vi "DHE_DRV_stop_sequence.vi"(11 "error in (no error)":errorcluster) -> (15 "error out":errorcluster)   [LabVIEW 2016]
doc: "This VI closes the I/O interface with the instrument."
uses:
  c/lib/libarcDHE.so
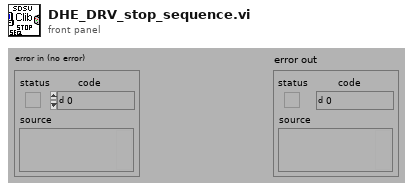
[diagram p1: front panel]
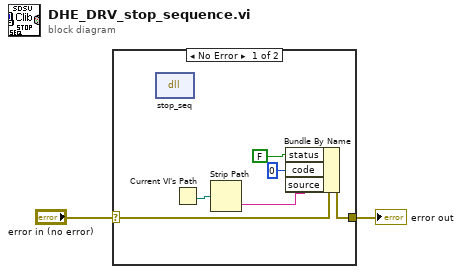
[diagram p0: block diagram]
diagram:
  n1 = case shown="No Error" "error in (no error)" {
    selector: "error in (no error)" -> [w5 w9]
    tunnel: [w6 w9] -> w2
    frame No Error {
      n2 = dll-call lib="home/simager/panview/PAN/Modules/SDSU/private/c/lib/libarcDHE.so" fn="stop_seq"() -> ()  [unwired: 3 in, 3 out]
      n3 = Current VI's Path() -> (path=w8:path)
      n4 = Strip Path(path=w8) -> (name=w7:string)  [unwired: 1 out]
      n5 = Bundle By Name(cluster=w5, "status"=FALSE, "code"=0, "source"=w7) -> (w6:errorcluster)
    }
    frame Error {
    }
  }
  "error out" <- w2
